vi "Write Periodic Delay Parameters.vi"(10 "Periodic Delay Parameters":cluster{"Range (ps)":i32, "Offset (ps)":i32}, 11 "Abstract Delay Line in":refnum<class "Abstract Delay Line.lvclass">) -> (3 "Abstract Delay Line out":refnum<class "Abstract Delay Line.lvclass">)   [LabVIEW 2016, in "_Delay Line.lvlib" / "Abstract Delay Line.lvclass"]
uses:
  Abstract Delay Line.lvclass
  Abstract Delay Line.lvclass/Abstract Delay Line.ctl
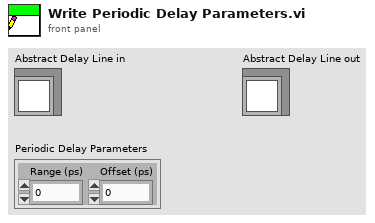
[diagram p1: front panel]
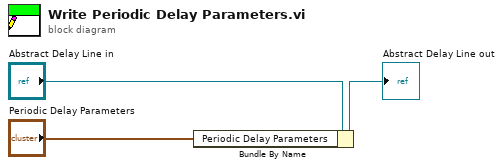
[diagram p0: block diagram]
diagram:
  n1 = Bundle By Name(cluster="Abstract Delay Line in", "Periodic Delay Parameters"="Periodic Delay Parameters") -> (→"Abstract Delay Line out":refnum<class "Abstract Delay Line.lvclass">)
